vi "Panel.vi"(8 "error in (no error)":errorcluster, 11 "ArrayBlank in":refnum<class "ArrayBlank.lvclass">) -> ()   [LabVIEW 2018, in "OOPanel.lvlib" / "ArrayBlank.lvclass"]
uses:
  ArrayBlank.lvclass
  C:/dev/source/Libraries/OOPanel/OOPanel/Panel/Panel.lvclass
  Panel/Panel.lvclass
types:
  T1 = typedef "OOPanel.lvlib/Panel.lvclass/Panel Events.ctl" = cluster{"Close":refnum<user-event>, "Visibility Changed":refnum<user-event>}
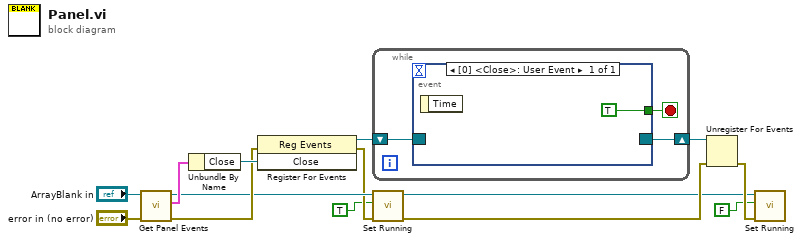
[diagram p0: block diagram]
diagram:
  n1 = call "Get Panel Events.vi"("error in (no error)"="error in (no error)", "Panel in"="ArrayBlank in") -> ("error out"=w10:errorcluster, "Panel Events"=w12:T1, "Panel out"=w9:refnum<class "ArrayBlank.lvclass">)  [unwired: 7 in]
  n2 = Unbundle By Name(w12) -> ("Close"=w11:refnum<user-event>)
  n3 = register-events(error in=w10, w11) -> (reference out=w6:refnum<event-registration>, error out=w8:errorcluster)  [unwired: 1 in]
  n4 = while {
    shift-right: [w16] -> w5
    shift-left: w6 -> [w17]
    stop <- w15 stop-if-true
    n5 = event shown="[0] <Close>: User Event" {
      selector: w17 -> [_]
      dyn-events: [_] -> w16
      timeout: _ -> [_]
      tunnel: [TRUE] -> w15
      event User Event {
        n6 = event-data() -> ()  [unwired: 1 in, 1 out]
      }
    }
  }
  n7 = call "Set Running.vi"("error in (no error)"=w8, "Running"=TRUE, "Panel in"=w9) -> ("error out"=w4:errorcluster, "Panel out"=w2:refnum<class "ArrayBlank.lvclass">)  [unwired: 7 in]
  n8 = Unregister For Events(event registration refnum=w5, error in=w4) -> (error out=w3:errorcluster)
  n9 = call "Set Running.vi"("error in (no error)"=w3, "Running"=FALSE, "Panel in"=w2) -> ()  [unwired: 7 in, 2 out]
